vi "DataProcessor_forAnalysis.vi"(5 "Data":dbl[][](array[numeric])) -> (0 "PumpOff":dbl[](array[numeric]), 1 "PumpOn":dbl[](array[numeric]), 2 "Raman":dbl[](array[numeric]))   [LabVIEW 2014]
panel:
  # "This vi takes the Data from the DataGrabber.vi and processes it splitting up the Raman Pump On and Off spectra as well as creating the Raman Gain Spectrum"
  # "Data Output"
  # "Data Input"
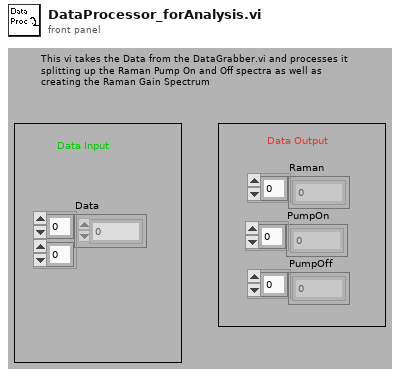
[diagram p1: front panel]
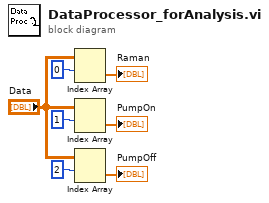
[diagram p0: block diagram]
diagram:
  n1 = Index Array(array="Data", index (row)=0) -> (element=→"Raman":dbl[])  [unwired: 1 in]
  n2 = Index Array(array="Data", index (row)=1) -> (element=→"PumpOn":dbl[])  [unwired: 1 in]
  n3 = Index Array(array="Data", index (row)=2) -> (element=→"PumpOff":dbl[])  [unwired: 1 in]
